vi "vicrypt_ppkg.vi"() -> (0 "Modulo":string, 1 "Private key":string, 2 "Public key":string)   [LabVIEW 2017]
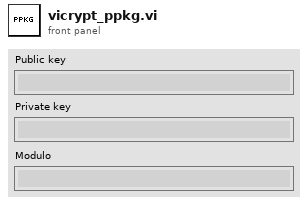
[diagram p1: front panel]
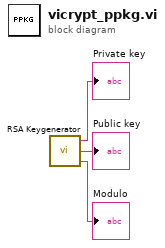
[diagram p0: block diagram]
diagram:
  n1 = call "RSA Keygenerator.vi"() -> ("Private Exponent (d)"=→"Private key":string, "Public Exponent (e)"=→"Public key":string, "Puplic Modulo (n)"=→"Modulo":string)  [unwired: 3 in, 2 out]
